vi "Autonomous Independent - Copy.vi"   [LabVIEW 2023]
doc: "This VI is called when autonomous begins, and will automatically be terminated when autonomous ends. You can carry out timed or sensor driven robot movement independently without needing to return to the caller."
uses:
  Arm2/ArmGetSetpointEnum.ctl
  <vilib>/Rock Robotics/Network Tables/NT Read String.vi
panel:
  # "Be sure to right-click and choose Data Operations>>Make Current Value default if you want to save the array values with the VI"
types:
  T1 = typedef "ArmGetSetpointEnum.ctl" = enum16{"ArmFloorPickup", "ArmAmpDeposit", "ArmSpeakerShoot", "ArmStartPosition", "ArmRestPosition", "ArmSourceIntake", "ArmAwayShoot"}
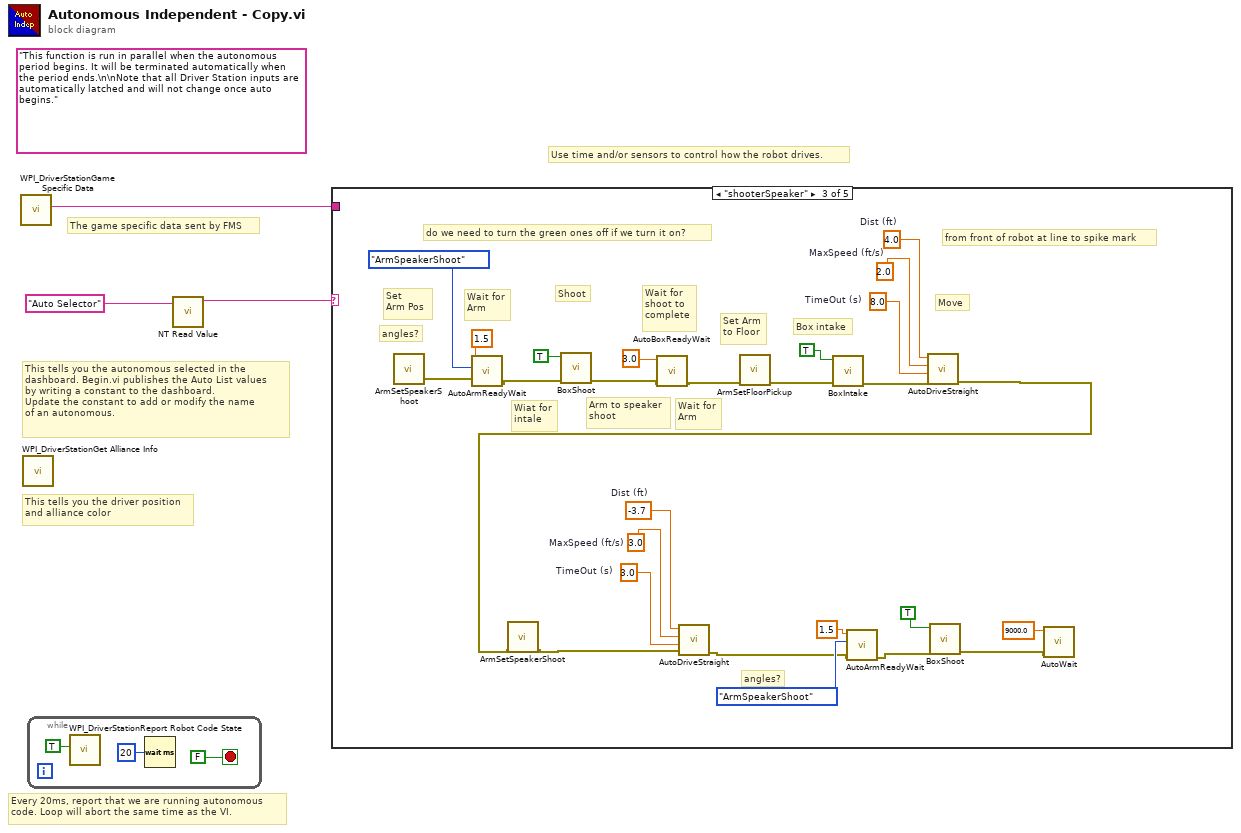
[diagram p0: block diagram]
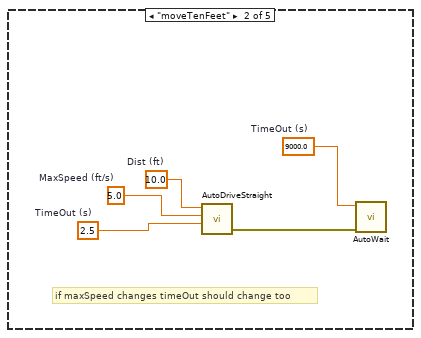
[diagram p3: hidden frame]
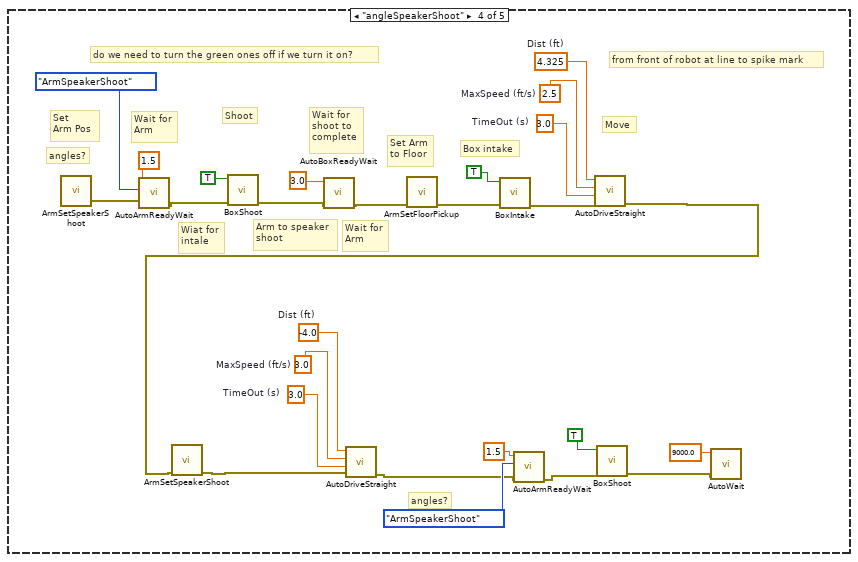
[diagram p4: hidden frame]
diagram:
  (unwired) "This function is run in parallel when the autonomous period begins. It will be terminated automatically when the period ends.\n\nNote that all Driver Station inputs are automatically latched and will not change once auto begins."
  # "The game specific data sent by FMS"
  # "This tells you the autonomous selected in the \ndashboard. Begin.vi publishes the Auto List values\nby writing a constant to the dashboard.\nUpdate the constant to add or modify the name\nof an autonomous."
  # "Every 20ms, report that we are running autonomous\ncode. Loop will abort the same time as the VI."
  # "Use time and/or sensors to control how the robot drives."
  # "This tells you the driver position\nand alliance color"
  n1 = call <vilib>:"WPI_DriverStationGame Specific Data.vi"() -> ("Game Specific Data"=w1:string)  [unwired: 11 in]
  n2 = call <vilib>:"WPI_DriverStationGet Alliance Info.vi"() -> ()  [unwired: 12 out]
  n3 = while {
    stop <- FALSE stop-if-true
    n4 = call <vilib>:"WPI_DriverStationReport Robot Code State.vi"("Autonomous"=TRUE) -> ()  [unwired: 10 in, 1 out]
    n5 = Wait (ms)(milliseconds to wait=u32 20) -> ()  [unwired: 1 out]
  }
  n6 = call-poly <vilib>:"NT Read Value.vi"("name"="Auto Selector" ("Name")) -> ("value"=w2:string)  [unwired: 8 in, 2 out]
  n7 = case shown="\"shooterSpeaker\"" w2 {
    tunnel: w1 -> [_ _ _ _ _]
    frame Default {
      # "You can put your main auto here, or you can right-click on the case and make any\nother frame be the default case."
      # "This is the frame that will execute if no selection is made, or if it is not recognized"
    }
    frame "moveTenFeet" {
      w7 = 9000.0  # TimeOut (s)
      w9 = 2.5  # TimeOut (s)
      w10 = 5.0  # MaxSpeed (ft/s)
      w11 = 10.0  # Dist (ft)
      # "if maxSpeed changes timeOut should change too"
      n8 = call "AutoDriveStraight.vi"("TimeOut (s)"=w9, "MaxSpeed (ft/s)"=w10, "Dist (ft)"=w11) -> ("error out"=w8:errorcluster)  [unwired: 8 in]
      n9 = call "AutoWait.vi"("error in (no error)"=w8, "TimeOut (s)"=w7) -> ()  [unwired: 9 in, 1 out]
    }
    frame "shooterSpeaker" {
      w15 = 3.0  # TimeOut (s)
      w16 = 3.0  # MaxSpeed (ft/s)
      w17 = -3.7  # Dist (ft)
      w34 = 8.0  # TimeOut (s)
      w35 = 2.0  # MaxSpeed (ft/s)
      w36 = 4.0  # Dist (ft)
      # "Wait for\nArm"
      # "Arm to speaker\nshoot"
      # "Wiat for\nintale"
      # "Box intake"
      # "Move"
      # "Set Arm\nto Floor"
      # "Wait for\nshoot to\ncomplete"
      # "Shoot"
      # "Wait for\nArm"
      # "Set\nArm Pos"
      # "do we need to turn the green ones off if we turn it on?"
      # "angles?"
      # "angles?"
      # "from front of robot at line to spike mark"
      n10 = call "ArmSetSpeakerShoot.vi"() -> ("error out"=w27:errorcluster)  [unwired: 11 in]
      n11 = call "AutoArmReadyWait.vi"("error in (no error)"=w27, "ArmSetpoints"=ArmGetSetpointEnum."ArmSpeakerShoot", "TimeOut (s)"=1.5) -> ("error out"=w26:errorcluster)  [unwired: 8 in]
      n12 = call "BoxShoot.vi"("error in (no error)"=w26, "Box shoot"=TRUE) -> ("error out"=w24:errorcluster)  [unwired: 9 in]
      n13 = call "AutoBoxReadyWait.vi"("error in (no error)"=w24, "TimeOut (s)"=3.0) -> ("error out"=w23:errorcluster)  [unwired: 9 in]
      n14 = call "ArmSetFloorPickup.vi"("error in (no error)"=w23) -> ("error out"=w29:errorcluster)  [unwired: 10 in]
      n15 = call "BoxIntake.vi"("error in (no error)"=w29, "Box intake"=TRUE) -> ("error out"=w28:errorcluster)  [unwired: 9 in]
      n16 = call "AutoDriveStraight.vi"("error in (no error)"=w28, "TimeOut (s)"=w34, "MaxSpeed (ft/s)"=w35, "Dist (ft)"=w36) -> ("error out"=w13:errorcluster)  [unwired: 7 in]
      n17 = call "ArmSetSpeakerShoot.vi"("error in (no error)"=w13) -> ("error out"=w12:errorcluster)  [unwired: 10 in]
      n18 = call "AutoDriveStraight.vi"("error in (no error)"=w12, "TimeOut (s)"=w15, "MaxSpeed (ft/s)"=w16, "Dist (ft)"=w17) -> ("error out"=w14:errorcluster)  [unwired: 7 in]
      n19 = call "AutoArmReadyWait.vi"("error in (no error)"=w14, "ArmSetpoints"=ArmGetSetpointEnum."ArmSpeakerShoot", "TimeOut (s)"=1.5) -> ("error out"=w21:errorcluster)  [unwired: 8 in]
      n20 = call "BoxShoot.vi"("error in (no error)"=w21, "Box shoot"=TRUE) -> ("error out"=w31:errorcluster)  [unwired: 9 in]
      n21 = call "AutoWait.vi"("error in (no error)"=w31, "TimeOut (s)"=9000.0) -> ()  [unwired: 9 in, 1 out]
    }
    frame "angleSpeakerShoot" {
      w41 = 3.0  # TimeOut (s)
      w42 = 3.0  # MaxSpeed (ft/s)
      w43 = -4.0  # Dist (ft)
      w60 = 3.0  # TimeOut (s)
      w61 = 2.5  # MaxSpeed (ft/s)
      w62 = 4.325  # Dist (ft)
      # "Wait for\nArm"
      # "Arm to speaker\nshoot"
      # "Wiat for\nintale"
      # "Box intake"
      # "Move"
      # "Set Arm\nto Floor"
      # "Wait for\nshoot to\ncomplete"
      # "Shoot"
      # "Wait for\nArm"
      # "Set\nArm Pos"
      # "do we need to turn the green ones off if we turn it on?"
      # "angles?"
      # "angles?"
      # "from front of robot at line to spike mark"
      n22 = call "ArmSetSpeakerShoot.vi"() -> ("error out"=w53:errorcluster)  [unwired: 11 in]
      n23 = call "AutoArmReadyWait.vi"("error in (no error)"=w53, "ArmSetpoints"=ArmGetSetpointEnum."ArmSpeakerShoot", "TimeOut (s)"=1.5) -> ("error out"=w52:errorcluster)  [unwired: 8 in]
      n24 = call "BoxShoot.vi"("error in (no error)"=w52, "Box shoot"=TRUE) -> ("error out"=w50:errorcluster)  [unwired: 9 in]
      n25 = call "AutoBoxReadyWait.vi"("error in (no error)"=w50, "TimeOut (s)"=3.0) -> ("error out"=w49:errorcluster)  [unwired: 9 in]
      n26 = call "ArmSetFloorPickup.vi"("error in (no error)"=w49) -> ("error out"=w55:errorcluster)  [unwired: 10 in]
      n27 = call "BoxIntake.vi"("error in (no error)"=w55, "Box intake"=TRUE) -> ("error out"=w54:errorcluster)  [unwired: 9 in]
      n28 = call "AutoDriveStraight.vi"("error in (no error)"=w54, "TimeOut (s)"=w60, "MaxSpeed (ft/s)"=w61, "Dist (ft)"=w62) -> ("error out"=w39:errorcluster)  [unwired: 7 in]
      n29 = call "ArmSetSpeakerShoot.vi"("error in (no error)"=w39) -> ("error out"=w38:errorcluster)  [unwired: 10 in]
      n30 = call "AutoDriveStraight.vi"("error in (no error)"=w38, "TimeOut (s)"=w41, "MaxSpeed (ft/s)"=w42, "Dist (ft)"=w43) -> ("error out"=w40:errorcluster)  [unwired: 7 in]
      n31 = call "AutoArmReadyWait.vi"("error in (no error)"=w40, "ArmSetpoints"=ArmGetSetpointEnum."ArmSpeakerShoot", "TimeOut (s)"=1.5) -> ("error out"=w47:errorcluster)  [unwired: 8 in]
      n32 = call "BoxShoot.vi"("error in (no error)"=w47, "Box shoot"=TRUE) -> ("error out"=w57:errorcluster)  [unwired: 9 in]
      n33 = call "AutoWait.vi"("error in (no error)"=w57, "TimeOut (s)"=9000.0) -> ()  [unwired: 9 in, 1 out]
    }
    frame "Your Turn" {
    }
  }
